vi "CRYStep Revert.vi"(9 "Proper VI No":u32) -> (2 "StepName":string, 3 "Flattened Step":string)   [LabVIEW 2013]
uses:
  CRYProject/CRYProject Editor Global.vi
panel:
  out "Category":string
  in  "Boolean":bool
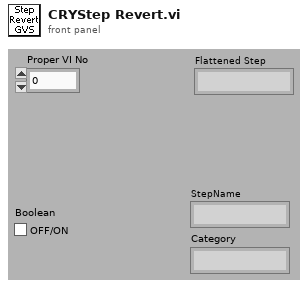
[diagram p1: front panel]
types:
  T1 = typedef "CRYStep.ctl" = cluster{"No.VI":i32, "Category":string, "StepName":string, "Seq setup flattened":string, "Comment":string, "Steps config.":bool[], "Jump config":i32[], "Start":dbl, "Increment":dbl, "Name":string, "Unit":string, "Y data":u16, "Y prefix":string, "Y dB ref":dbl, "Y unit":string, "Repeat State Array":cluster{"Start":dbl, "Increment":dbl, "Count":i32, "Num":i32}[]}
  T2 = cluster{"Content":string, "Name":string, "Level":u32, "Category":string}[]
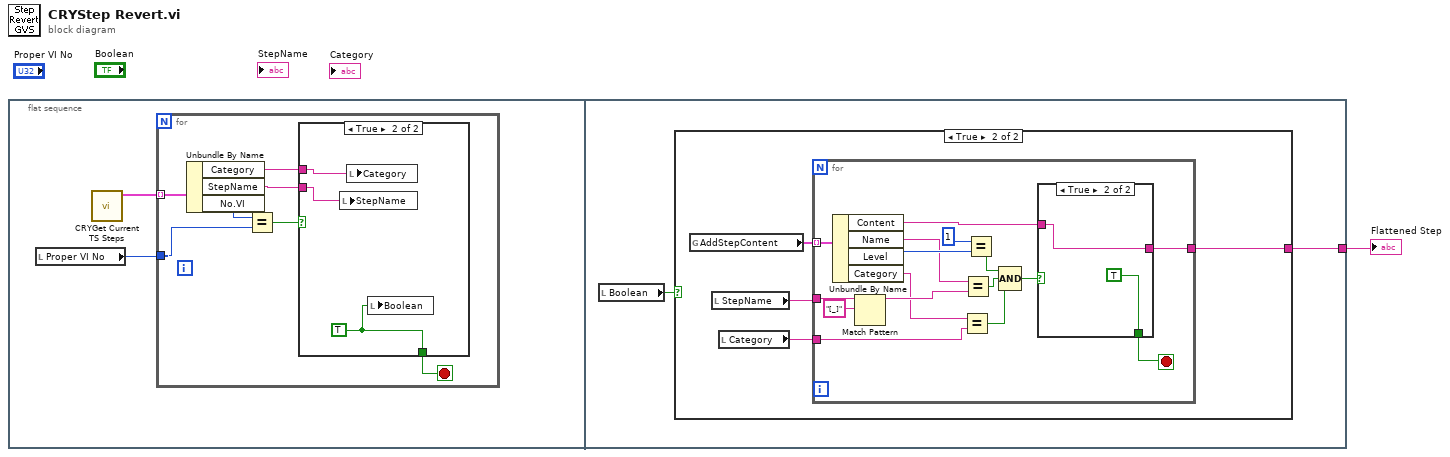
[diagram p0: block diagram]
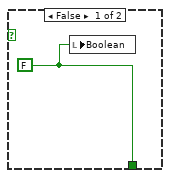
[diagram p2: hidden frame]
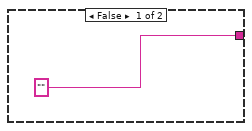
[diagram p3: hidden frame]
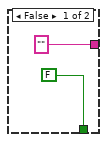
[diagram p4: hidden frame]
diagram:
  n1 = flat-sequence {
    tunnel: [w15] -> w1
    frame #0 {
      n2 = local read "Proper VI No"() -> (w3:u32)
      n3 = call "CRYGet Current TS Steps.vi"() -> ("Steps"=w2:T1[])  [unwired: 7 in, 4 out]
      n4 = for {
        tunnel: w2 -> [w10] mode=indexing
        tunnel: w3 -> [w8]
        stop <- w5 stop-if-true
        n5 = Unbundle By Name(w10) -> ("Category"=w4:string, "StepName"=w6:string, "No.VI"=w9:i32)
        n6 = Equal?(x=w9, y=w8) -> (x = y?=w7:bool)
        n7 = case shown="True" w7 {
          tunnel: w6 -> [_ w13]
          tunnel: [w11 w14] -> w5
          tunnel: w4 -> [_ w12]
          frame False {
            w11 = FALSE
            n8 = local write "Boolean"(w11) -> ()
          }
          frame True {
            w14 = TRUE
            n9 = local write "StepName"(w13) -> ()
            n10 = local write "Category"(w12) -> ()
            n11 = local write "Boolean"(w14) -> ()
          }
        }
      }
    }
    frame #1 {
      n12 = local read "Boolean"() -> (w16:bool)
      n13 = case shown="True" w16 {
        tunnel: ["" ("String") w20] -> w15
        frame False {
        }
        frame True {
          n14 = global read "CRYProject Editor Global.vi" "AddStepContent"() -> (w19:T2)
          n15 = local read "StepName"() -> (w21:string)
          n16 = local read "Category"() -> (w18:string)
          n17 = for {
            tunnel: w21 -> [w27]
            tunnel: [w32] -> w20
            tunnel: w19 -> [w31] mode=indexing
            tunnel: w18 -> [w23]
            stop <- w33 stop-if-true
            n18 = Unbundle By Name(w31) -> ("Content"=w28:string, "Name"=w29:string, "Level"=w30:u32, "Category"=w24:string)
            n19 = Match Pattern(string=w27, regular expression="[_]") -> (before substring=w25:string)  [unwired: 4 out]
            n20 = Equal?(x=w24, y=w23) -> (x = y?=w22:bool)
            n21 = Equal?(x=w29, y=w25) -> (x = y?=w37:bool)
            n22 = Equal?(x=1 ("y"), y=w30) -> (x = y?=w36:bool)
            n23 = Compound Arithmetic op=AND(w36, w37, w22) -> (w35:bool)
            n24 = case shown="True" w35 {
              tunnel: [FALSE TRUE] -> w33
              tunnel: ["" ("String") w40] -> w32
              tunnel: w28 -> [_ w40]
              frame False {
              }
              frame True {
              }
            }
          }
        }
      }
    }
  }
  "Flattened Step" <- w1
